vi "Bernards_2_2400.vi"() -> ()   [LabVIEW 2018]
uses:
  <vilib>/Utility/file.llb/Write Delimited Spreadsheet (string).vi
  <instrlib>/Keithley 24XX/Public/Data/Read (Single Point).vi
  <instrlib>/Keithley 24XX/Keithley 24XX.lvlib
  <vilib>/Analysis/NI_AALBase.lvlib
panel:
  in  "Auto (up)\nUser (down)":bool
  in  "User Selected":dbl[](array[numeric])=[-2e-08, -5e-08, -1e-07]
  in  "CC (on), CV (off)":bool
  out "Current (A) 2":dbl format="%.2e"
  out "error 8":string
  in  "Keithley 2401 (new)\nVISA resource #2 = 22":refnum<visa-resource-name>="GPIB0::22::INSTR"
  in  "Delay Gate (s) 2":dbl=60.0 format="%#.3g"
  in  "source/measure (V/I:0)":u16(ring)=1 items=["voltage/current", "current/voltage"]
  out "Setpoint Array":dbl[](array[numeric])=[-2e-08, -5e-08, -1e-07]
  in  "Measurement Speed (1 PLC)":dbl=1.0 format="%.2g"
  in  "Initial Gate Setting":dbl=1e-08 format="%#.3e"
  in  "Voltage Compliance Limit 2401 (V)":dbl=-0.95 format="%#.3f"
  in  "Current Compliance\nLimit 2401 (A)":dbl=0.10000000009313226
  in  "Delay Gate (s)":dbl=30.0 format="%#.3g"
  in  "Keithley 237 GPIB address":string="17"
  in  "Wait Time Btwn Keithley Readings (ms)":i32=30
  out "Time Btwn Iterations (ms)":i32
  out "Total Elapsed Time (ms)":i32
  out "# Avgs":i32
  out "Current (A)":dbl format="%.2e"
  in  "Total Measure Time (s)":dbl=210.0 format="%#.3g"
  in  "Drain Bias (V)":dbl=-0.6 format="%#.3g"
  in  "Current Compliance\nLimit (A)":dbl=0.5 format="%#.3e"
  in  "Keithley 2400 (old)\nVISA resource #1 = 24":refnum<visa-resource-name>="GPIB0::24::INSTR"
  in  "ApproximateTime Step (ms)":dbl=300.0 format="%#.3g"
  in  "Current Offset":dbl format="%^#_3e"
  out "I-t Measurement\nBy M. Ziffer 7/3/2014":cluster{dbl[], dbl[]}(graph)={[-2.0, -1.95, -1.9, -1.85, -1.8, -1.75, -1.7, -1.65, -1.6, -1.55, -1.5, -1.45, -1.4, -1.35, -1.2999999999999998, -1.25, -1.2, -1.15, -1.1, -1.0499999999999998, -1.0, -0.95, -0.8999999999999999, -0.8499999999999999, -0.7999999999999998, -0.75, -0.7, -0.6499999999999999, -0.5999999999999999, -0.5499999999999998, -0.5, -0.44999999999999996, -0.3999999999999999, -0.34999999999999987, -0.2999999999999998, -0.25, -0.19999999999999996, -0.1499999999999999, -0.09999999999999987, -0.04999999999999982, 0.0, 0.050000000000000266, 0.10000000000000009, 0.1499999999999999, 0.20000000000000018, 0.25, 0.30000000000000027, 0.3500000000000001, 0.40000000000000036, 0.4500000000000002, 0.5, 0.5500000000000003, 0.6000000000000001, 0.6500000000000004, 0.7000000000000002, 0.75, 0.8000000000000003, 0.8500000000000001, 0.9000000000000004, 0.9500000000000002, 1.0, 1.0500000000000003, 1.1, 1.1500000000000004, 1.2000000000000002, 1.25, 1.3000000000000003, 1.35, 1.4000000000000004, 1.4500000000000002, 1.5, 1.5500000000000003, 1.6, 1.6500000000000004, 1.7000000000000002, 1.75, 1.8000000000000003, 1.85, 1.9000000000000004, 1.9500000000000002, 2.0, 1.95, 1.9, 1.85, 1.8, 1.75, 1.7, 1.65, 1.6, 1.55, 1.5, 1.45, 1.4, 1.35, 1.2999999999999998, 1.25, 1.2, 1.15, 1.1, 1.0499999999999998, 1.0, 0.95, 0.8999999999999999, 0.8499999999999999, 0.7999999999999998, 0.75, 0.7, 0.6499999999999999, 0.5999999999999999, 0.5499999999999998, 0.5, 0.44999999999999996, 0.3999999999999999, 0.34999999999999987, 0.2999999999999998, 0.25, 0.19999999999999996, 0.1499999999999999, 0.09999999999999987, 0.04999999999999982, 0.0, -0.050000000000000266, -0.10000000000000009, -0.1499999999999999, -0.20000000000000018, -0.25, -0.30000000000000027, -0.3500000000000001, -0.40000000000000036, -0.4500000000000002, -0.5, -0.5500000000000003, -0.6000000000000001, -0.6500000000000004, -0.7000000000000002, -0.75, -0.8000000000000003, -0.8500000000000001, -0.9000000000000004, -0.9500000000000002, -1.0, -1.0500000000000003, -1.1, -1.1500000000000004, -1.2000000000000002, -1.25, -1.3000000000000003, -1.35, -1.4000000000000004, -1.4500000000000002, -1.5, -1.5500000000000003, -1.6, -1.6500000000000004, -1.7000000000000002, -1.75, -1.8000000000000003, -1.85, -1.9000000000000004, -1.9500000000000002, -2.0], [-0.9617289445307117, -0.9618513744908972, -0.9601574911889584, -0.9603488957746004, -0.9598860982876659, -0.9595594700613103, -0.9590290885663679, -0.9586886097902229, -0.9580144940757807, -0.9570474587019399, -0.9571418538143588, -0.9562287187728303, -0.9551771894828052, -0.9535572870291384, -0.9535421571112963, -0.9533114258642045, -0.9520938012261039, -0.9513117179729429, -0.9508812384355169, -0.9504840780921618, -0.9504173840793213, -0.9482281628421478, -0.9464640811713977, -0.9453356785488072, -0.9439408336230415, -0.9428695575652444, -0.9416178906119992, -0.9396031084275935, -0.9378375248899987, -0.9354517815949719, -0.9324159524550173, -0.928767917889437, -0.9245502864168607, -0.9203528467096396, -0.9146985405384399, -0.908595454304189, -0.9012966039381313, -0.8917361646028689, -0.8808115851751085, -0.8684870433493713, -0.853007079283089, -0.8360736418594031, -0.8154860511533626, -0.7920970894092216, -0.7641180332150388, -0.7294003786125389, -0.6854183749419586, -0.6263231964633708, -0.5399961516707377, -0.4044042921440459, -0.19129744134883978, 0.11936942255465804, 0.5420583260977958, 1.0996962734707192, 1.8318907919106253, 2.7834859177196174, 3.9948214605959804, 5.494887344369723, 7.293988211209965, 9.39251059714275, 11.765998658717283, 14.371720946722268, 17.153138293174568, 20.070768287470067, 23.082285540692517, 26.15604905590766, 29.26009131920428, 32.38734131897913, 35.54092126952808, 38.70923397757575, 41.89103456238207, 45.09512285116253, 48.318234786641504, 51.57411300669423, 54.84161623237131, 58.130390342544004, 61.4596508891188, 64.79419021952893, 68.17503711098149, 71.57587551887687, 75.0023346626475, 71.8977923333163, 68.72637799211101, 65.51757272894447, 62.2950059155054, 59.076872390492845, 55.84672949319313, 52.615591470047114, 49.383497814590335, 46.15858586388574, 42.93308596012382, 39.714879010509975, 36.494540522470736, 33.276879251143754, 30.087779593472593, 26.903443634933772, 23.758388169345494, 20.669969771208738, 17.671195580039395, 14.804861569698371, 12.12778391916459, 9.68736655227705, 7.528128139792144, 5.673530623057721, 4.128839936603901, 2.8787577310032053, 1.895544581260216, 1.1383875896205915, 0.5622048852612092, 0.12746496878202787, -0.18928305409978952, -0.4042961076690051, -0.5411369085387429, -0.6286316214282486, -0.6871327837574404, -0.7298882072135505, -0.7640718647157413, -0.7921132761963248, -0.8155779431543743, -0.8358809022810104, -0.8523300154596555, -0.8668520109778625, -0.8802307520791266, -0.8907705198464766, -0.8998007445608903, -0.9078572589377096, -0.9150023626386364, -0.9215738644543149, -0.925261336930741, -0.9288795566582202, -0.9332418679701618, -0.9352489739462505, -0.9376688708058178, -0.9394550911063516, -0.9405290371496502, -0.9430050037047499, -0.9440335043698243, -0.9453382929096107, -0.9473152502994113, -0.9474565926568992, -0.9494901203645137, -0.94896546821346, -0.9503187058651598, -0.9511280452203158, -0.9523093469306558, -0.9532668704811476, -0.9541692143312739, -0.9545545822386634, -0.955485183435348, -0.9561708134622656, -0.956805602515258, -0.9577699122788996, -0.9578049002139094, -0.9580356870856992, -0.958780001168953, -0.9592832934359943, -0.9588639388381576, -0.959203916992021, -0.9603773199952523, -0.9611007191920772, -0.9623172869609168]}
  in  "First bias settle (ms)":dbl=2000.0 format="%#.2f"
  out "Outputfile":path
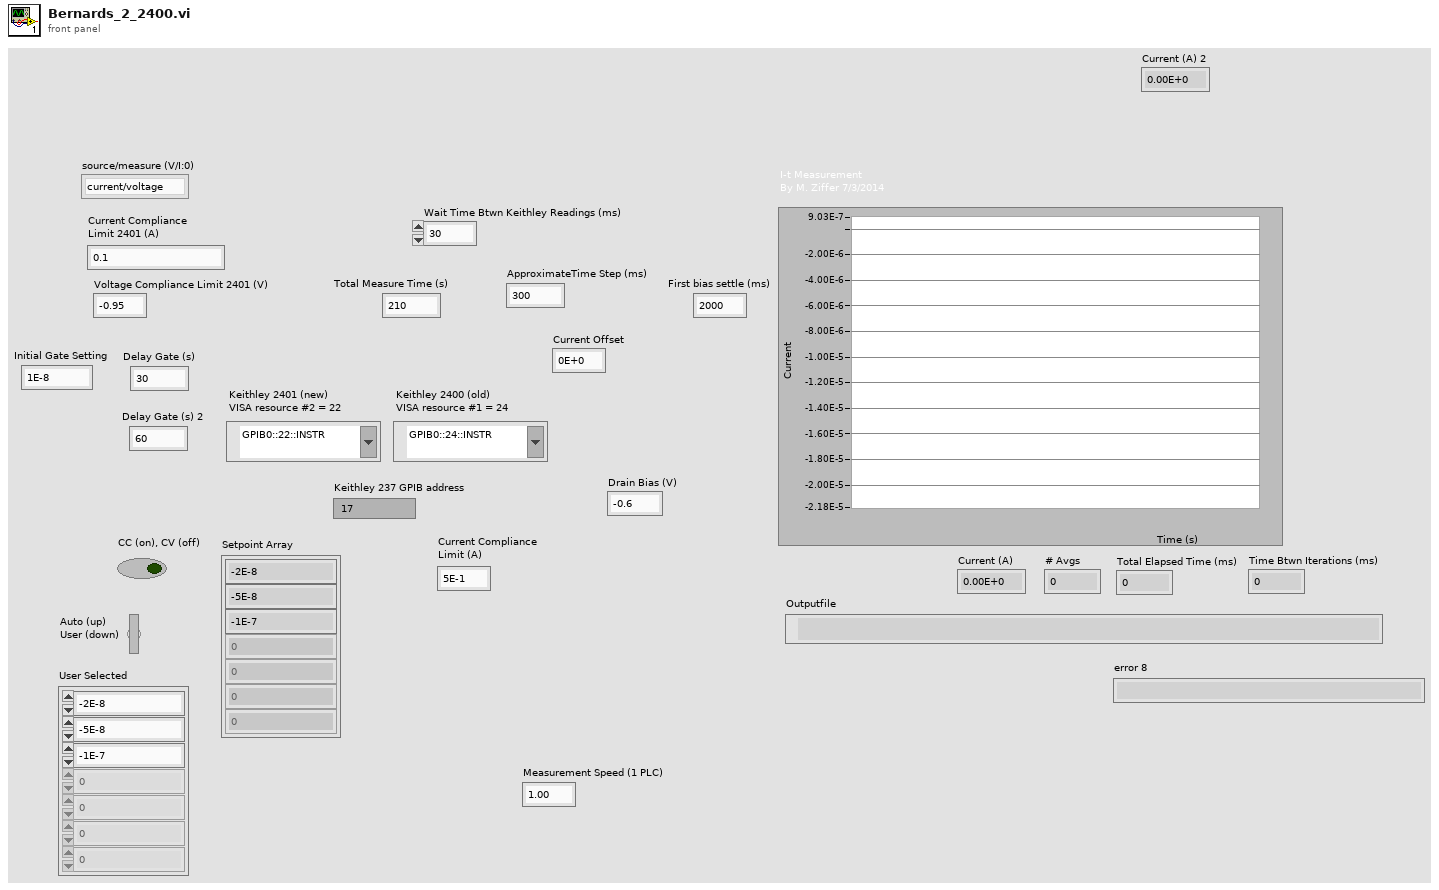
[diagram p1: front panel]
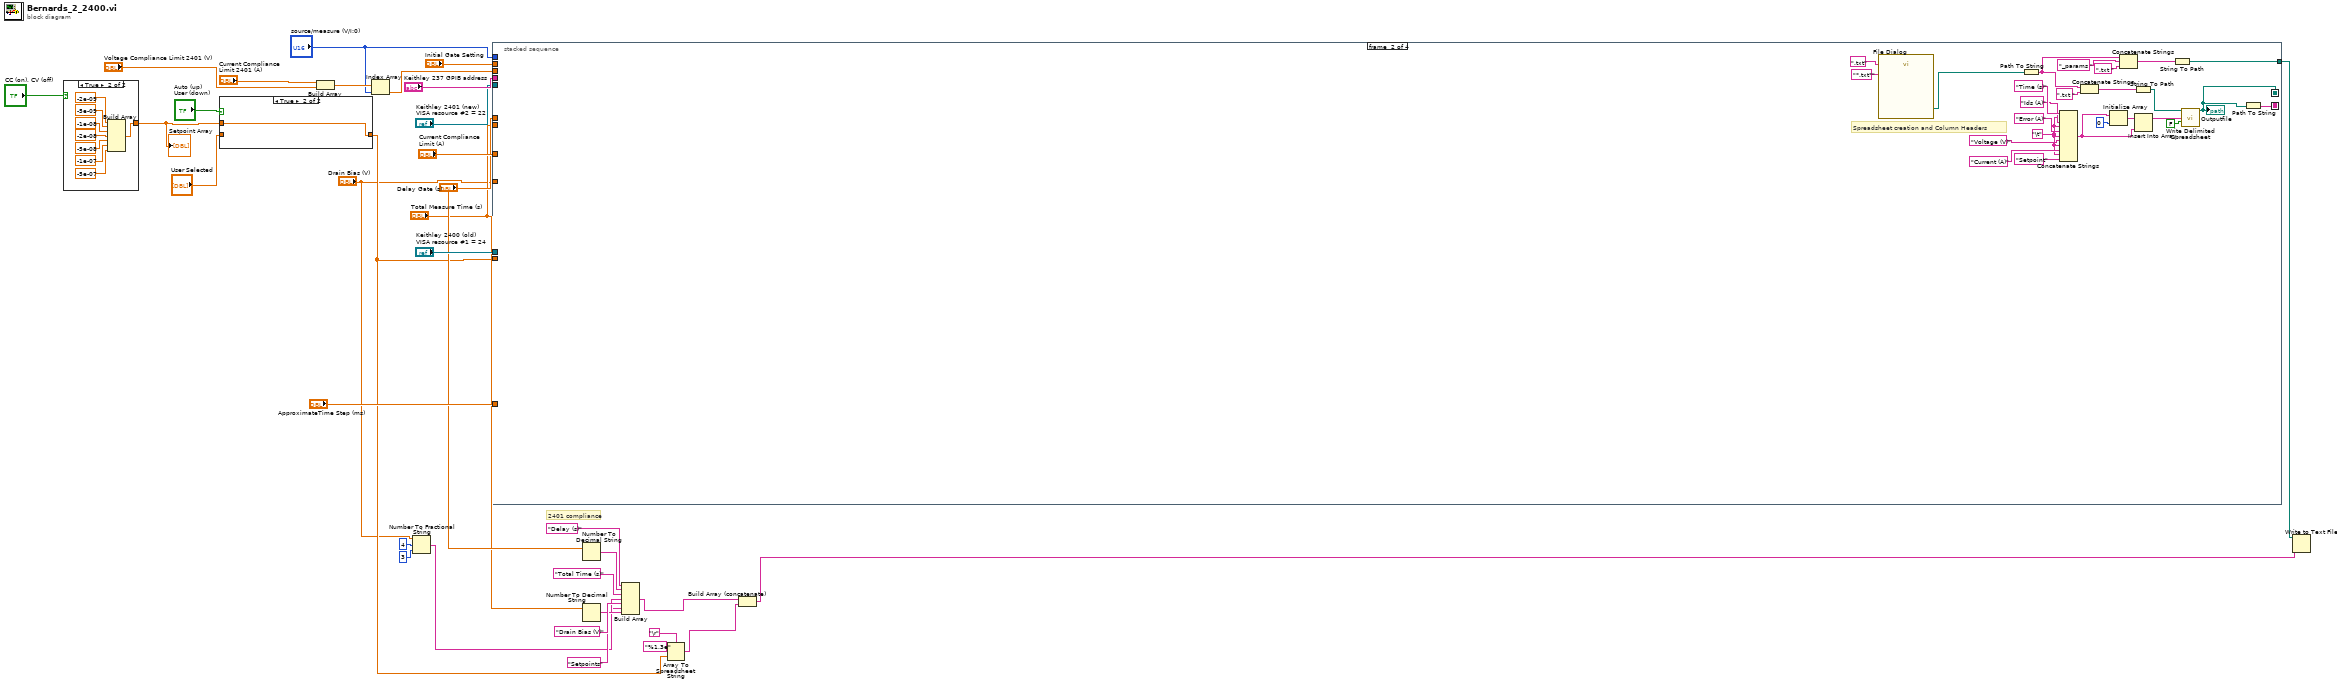
[diagram p0: block diagram]
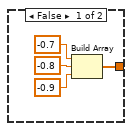
[diagram p3: hidden frame]
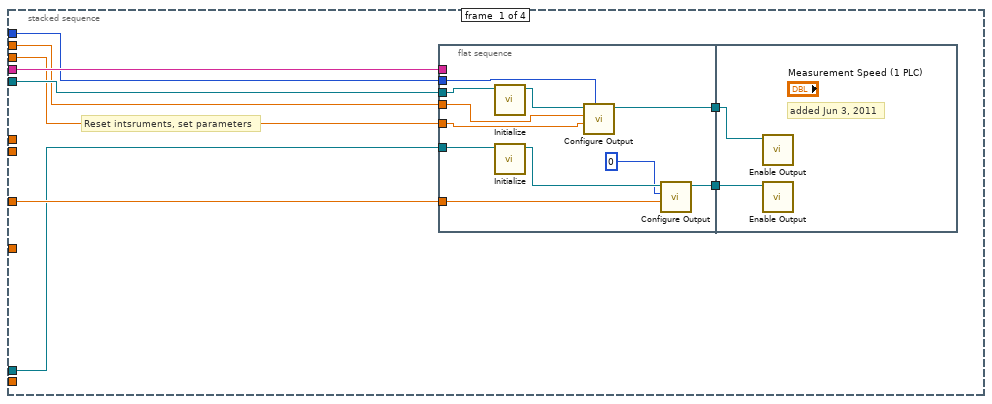
[diagram p4: hidden frame]
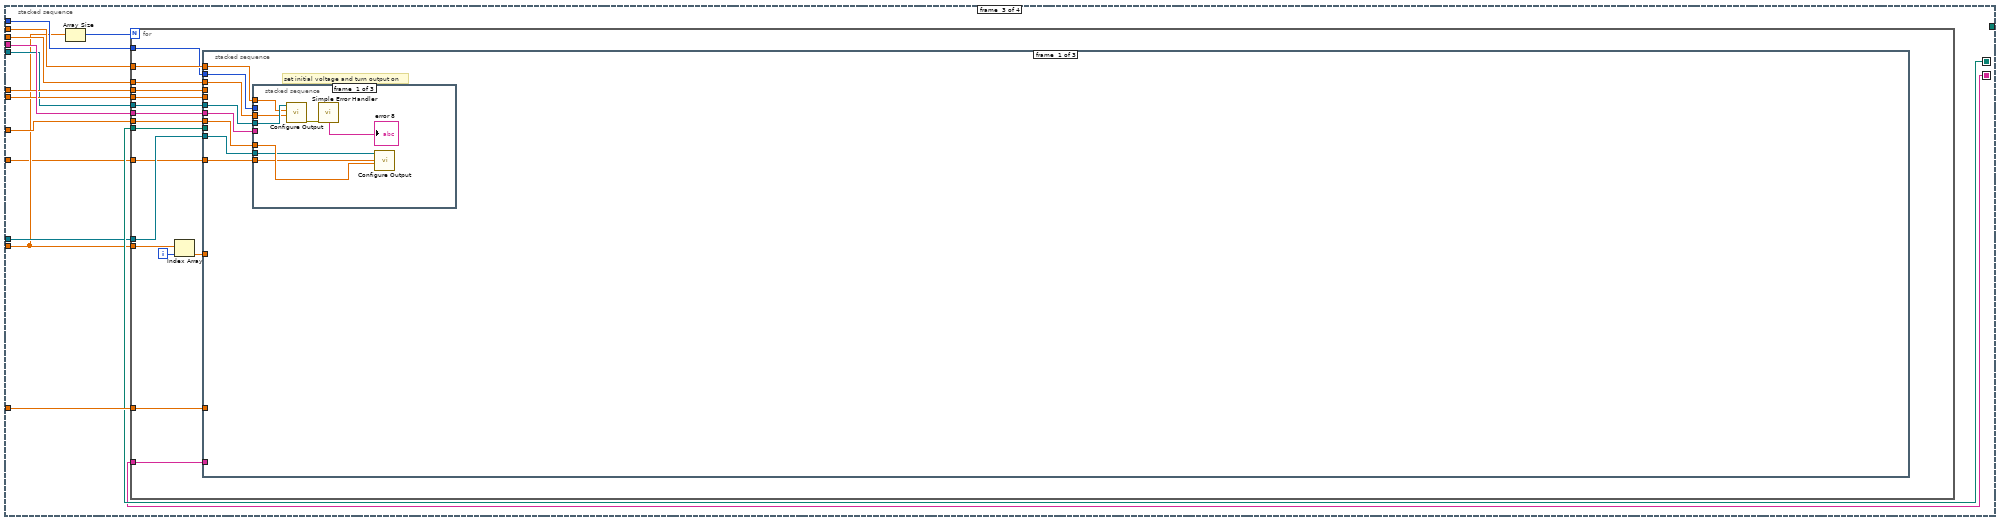
[diagram p5: hidden frame]
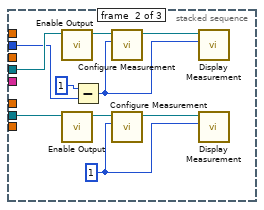
[diagram p6: hidden frame]
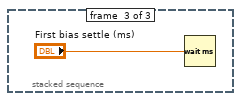
[diagram p7: hidden frame]
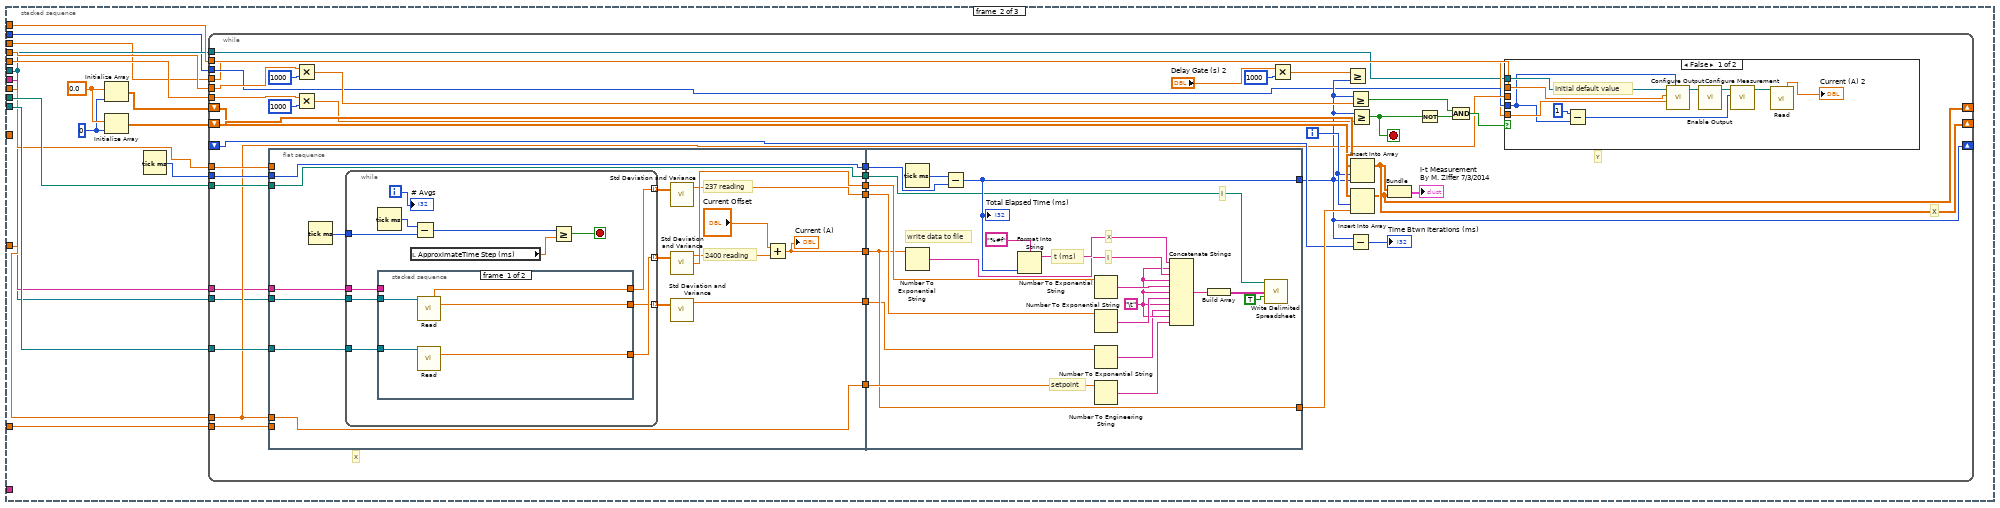
[diagram p8: hidden frame]
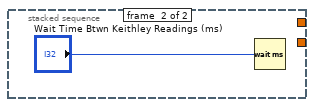
[diagram p9: hidden frame]
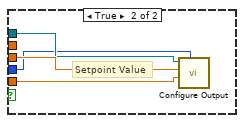
[diagram p10: hidden frame]
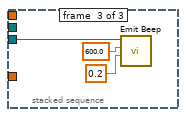
[diagram p11: hidden frame]
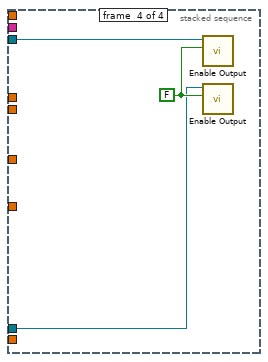
[diagram p12: hidden frame]
diagram:
  # "2401 compliance"
  n1 = case shown="True" "CC (on), CV (off)" {
    tunnel: [w38 w39] -> w17
    frame False {
      n2 = Build Array(-0.7, -0.8, -0.9) -> (w38:dbl[])
    }
    frame True {
      n3 = Build Array(-2e-09, -5e-09, -1e-08, -2e-08, -5e-08, -1e-07, -5e-07) -> (w39:dbl[])
    }
  }
  "Setpoint Array" <- w17
  n4 = case shown="True" "Auto (up)\nUser (down)" {
    tunnel: "User Selected" -> [w47 _]
    tunnel: w17 -> [_ w48]
    tunnel: [w47 w48] -> w16
    frame False {
    }
    frame True {
    }
  }
  n5 = Build Array("Current Compliance\nLimit 2401 (A)", "Voltage Compliance Limit 2401 (V)") -> (w24:dbl[])
  n6 = Index Array(array=w24, index="source/measure (V/I:0)") -> (element=w22:dbl)
  n7 = Number To Fractional String(number="Drain Bias (V)", width (-)=4, precision (6)=3) -> (F-format string=w3:string)  [unwired: 1 in]
  n8 = stacked-sequence {
    seq-local: [_ w76 _ _] -> [_ _ w109 _]
    seq-local: [_ w95 _ _] -> [_ _ w108 _]
    tunnel: "ApproximateTime Step (ms)" -> [_ _ w110 _]
    tunnel: "Keithley 2400 (old)\nVISA resource #1 = 24" -> [w56 _ w106 w284]
    tunnel: "Current Compliance\nLimit (A)" -> [w57 _ w107 _]
    tunnel: "Keithley 237 GPIB address" -> [w55 _ w104 _]
    tunnel: "Initial Gate Setting" -> [w51 _ w105 _]
    tunnel: "source/measure (V/I:0)" -> [w54 _ w99 _]
    tunnel: [_ w71 _ _] -> w30
    tunnel: "Delay Gate (s)" -> [_ _ w102 _]
    tunnel: "Total Measure Time (s)" -> [_ _ w101 _]
    tunnel: "Keithley 2401 (new)\nVISA resource #2 = 22" -> [w53 _ w100 w285]
    tunnel: w22 -> [w52 _ w98 _]
    tunnel: w16 -> [_ _ w97 _]
    tunnel: "Drain Bias (V)" -> [_ _ w96 _]
    frame #0 {
      # "Reset intsruments, set parameters"
      n9 = flat-sequence {
        tunnel: w56 -> [w67]
        tunnel: w57 -> [w63]
        tunnel: w55 -> [_]
        tunnel: w54 -> [w62]
        tunnel: w53 -> [w65]
        tunnel: w52 -> [w61]
        tunnel: w51 -> [w60]
        tunnel: [w68] -> w50
        tunnel: [w58] -> w49
        tunnel: w50 -> [w70]
        tunnel: w49 -> [w69]
        frame #0 {
          n10 = call <instrlib>:"Initialize.vi"("VISA resource name"=w65) -> ("VISA resource name out"=w64:refnum<visa-resource-name>)  [unwired: 9 in, 1 out]
          n11 = call <instrlib>:"Initialize.vi"("VISA resource name"=w67) -> ("VISA resource name out"=w66:refnum<visa-resource-name>)  [unwired: 9 in, 1 out]
          n12 = call <instrlib>:"Configure Output.vi"("Source Mode  (0: Voltage)"=w62, "Compliance  Level (0.1)"=w61, "Output Level (0)"=w60, "VISA resource name"=w64) -> ("VISA resource name out"=w58:refnum<visa-resource-name>)  [unwired: 2 in, 5 out]
          n13 = call <instrlib>:"Configure Output.vi"("Compliance  Level (0.1)"=w63, "Output Level (0)"=0, "VISA resource name"=w66) -> ("VISA resource name out"=w68:refnum<visa-resource-name>)  [unwired: 3 in, 5 out]
        }
        frame #1 {
          # "added Jun 3, 2011"
          n14 = call <instrlib>:"Enable Output.vi"("VISA resource name"=w69) -> ()  [unwired: 2 in, 9 out]
          n15 = call <instrlib>:"Enable Output.vi"("VISA resource name"=w70) -> ()  [unwired: 2 in, 9 out]
        }
      }
    }
    frame #1 {
      w78 = "\t"
      # "Spreadsheet creation and Column Headers"
      n16 = call "File Dialog"("default name"=".txt", "pattern (all files)"="*.txt*") -> ("selected path"=w82:path)  [unwired: 5 in, 8 out]
      n17 = Path To String(path=w82) -> (string=w73:string)
      n18 = Concatenate Strings("Time (s)", w78, "Ids (A)", w78, "Error (A)", w78, "Voltage (V)", w78, "Current (A)", w78, "Setpoint") -> (w93:string)
      n19 = Concatenate Strings(w73, ".txt " ("string")) -> (w81:string)
      n20 = Initialize Array(w93, 0 ("dimension size")) -> (w92:string[])
      n21 = Concatenate Strings(w73, "_params " ("string"), ".txt " ("string")) -> (w72:string)
      n22 = String To Path(string=w81) -> (path=w80:path)
      n23 = Insert Into Array(array=w92, new element=w93) -> (w85:string[])  [unwired: 1 in]
      n24 = String To Path(string=w72) -> (path=w71:path)
      n25 = call-poly <vilib>:"Write Delimited Spreadsheet.vi"("file path (dialog if empty)"=w80, "1D data"=w85, "append to file? (new file:F)"=FALSE) -> ("new file path (Not A Path if cancelled)"=w76:path)  [unwired: 11 in, 1 out]
      "Outputfile" <- w76
      n26 = Path To String(path=w76) -> (string=w95:string)
    }
    frame #2 {
      n27 = Array Size(array=w97) -> (size(s)=w103:i32)
      n28 = for {
        N: w103 -> [_]
        tunnel: w110 -> [w126]
        tunnel: w109 -> [w125]
        tunnel: w108 -> [w124]
        tunnel: w107 -> [w123]
        tunnel: w106 -> [w122]
        tunnel: w105 -> [w121]
        tunnel: w104 -> [w115]
        tunnel: w97 -> [w120]
        tunnel: w102 -> [w117]
        tunnel: w101 -> [w116]
        tunnel: w100 -> [w114]
        tunnel: w99 -> [w113]
        tunnel: w98 -> [w112]
        tunnel: w96 -> [w111]
        i -> [w118]
        n29 = Index Array(array=w120, index=w118) -> (element=w119:dbl)
        n30 = stacked-sequence {
          tunnel: w126 -> [_ w163 _]
          tunnel: w125 -> [_ w170 _]
          tunnel: w124 -> [_ _ _]
          tunnel: w123 -> [w134 w164 _]
          tunnel: w122 -> [w133 w165 w283]
          tunnel: w121 -> [w130 w161 _]
          tunnel: w115 -> [w132 w157 _]
          tunnel: w119 -> [_ w160 _]
          tunnel: w117 -> [_ w159 _]
          tunnel: w116 -> [_ w158 _]
          tunnel: w114 -> [w131 w156 _]
          tunnel: w113 -> [w129 w155 _]
          tunnel: w112 -> [w128 w154 _]
          tunnel: w111 -> [w127 _ _]
          frame #0 {
            # "set initial voltage and turn output on"
            n31 = stacked-sequence {
              tunnel: w133 -> [w141 w152 _]
              tunnel: w134 -> [w142 _ _]
              tunnel: w132 -> [_ _ _]
              tunnel: w131 -> [w140 w151 _]
              tunnel: w130 -> [w139 _ _]
              tunnel: w129 -> [_ w147 _]
              tunnel: w128 -> [w138 _ _]
              tunnel: w127 -> [w135 _ _]
              frame #0 {
                n32 = call <instrlib>:"Configure Output.vi"("Compliance  Level (0.1)"=w138, "Output Level (0)"=w139, "VISA resource name"=w140) -> ("error out"=w137:errorcluster)  [unwired: 3 in, 5 out]
                n33 = call <vilib>:"Simple Error Handler.vi"("error in (no error)"=w137) -> ("message"=→"error 8":string)  [unwired: 1 in, 7 out]
                n34 = call <instrlib>:"Configure Output.vi"("Compliance  Level (0.1)"=w142, "Output Level (0)"=w135, "VISA resource name"=w141) -> ()  [unwired: 3 in, 6 out]
              }
              frame #1 {
                w143 = 1
                n35 = call <instrlib>:"Enable Output.vi"("VISA resource name"=w151) -> ("VISA resource name out"=w150:refnum<visa-resource-name>)  [unwired: 2 in, 8 out]
                n36 = call <instrlib>:"Enable Output.vi"("VISA resource name"=w152) -> ("VISA resource name out"=w149:refnum<visa-resource-name>)  [unwired: 2 in, 8 out]
                n37 = Subtract(x=1, y=w147) -> (x-y=w144:i32)
                n38 = call <instrlib>:"Configure Measurement.vi"("Function (0: Volts)"=w144, "VISA resource name"=w150) -> ("VISA resource name out"=w145:refnum<visa-resource-name>)  [unwired: 8 in, 1 out]
                n39 = call <instrlib>:"Configure Measurement.vi"("Function (0: Volts)"=w143, "VISA resource name"=w149) -> ("VISA resource name out"=w146:refnum<visa-resource-name>)  [unwired: 8 in, 1 out]
                n40 = call <instrlib>:"Display Measurement.vi"("Displayed Measurement (0: Voltage)"=w144, "VISA resource name"=w145) -> ()  [unwired: 8 in, 2 out]
                n41 = call <instrlib>:"Display Measurement.vi"("Displayed Measurement (0: Voltage)"=w143, "VISA resource name"=w146) -> ()  [unwired: 8 in, 2 out]
              }
              frame #2 {
                n42 = Wait (ms)(milliseconds to wait="First bias settle (ms)") -> ()  [unwired: 1 out]
              }
            }
          }
          frame #1 {
            w166 = 0
            w167 = 0.0
            n43 = Initialize Array(w167, w166) -> (w168:dbl[])
            n44 = Initialize Array(w167, w166) -> (w169:dbl[])
            n45 = Tick Count (ms)() -> (millisecond timer value=w162:u32)
            n46 = while {
              shift-left: w168 -> [w209]
              shift-right: [w204] -> _
              shift-left: w169 -> [w210]
              shift-right: [w206] -> _
              tunnel: w170 -> [w211]
              tunnel: w165 -> [w208]
              tunnel: w164 -> [w207]
              tunnel: w163 -> [w202]
              tunnel: w162 -> [w197]
              shift-right: [w179] -> _
              shift-left: _ -> [w201]
              tunnel: w157 -> [w188]
              tunnel: w161 -> [w194]
              tunnel: w160 -> [w189]
              tunnel: w159 -> [w176]
              tunnel: w158 -> [w175]
              tunnel: w156 -> [w174]
              tunnel: w156 -> [w171]
              tunnel: w155 -> [w173]
              tunnel: w154 -> [w172]
              i -> [w203]
              stop <- w193 stop-if-true
              # "X"
              # "X"
              # "Y"
              n47 = flat-sequence {
                tunnel: w211 -> [w222]
                tunnel: [w222] -> w187
                tunnel: w208 -> [w216]
                tunnel: w207 -> [_]
                tunnel: w202 -> [_]
                tunnel: w197 -> [w221]
                tunnel: [w221] -> w186
                tunnel: w189 -> [w220]
                tunnel: [w220] -> w185
                tunnel: w188 -> [w223]
                tunnel: [w228] -> w184
                tunnel: [w224] -> w183
                tunnel: [w219] -> w182
                tunnel: [w218] -> w177
                tunnel: w174 -> [w217]
                tunnel: [w252] -> w205
                tunnel: w187 -> [w247]
                tunnel: w186 -> [w259]
                tunnel: [w258] -> w179
                tunnel: w185 -> [w255]
                tunnel: w184 -> [w261]
                tunnel: w183 -> [w252]
                tunnel: w182 -> [w254]
                tunnel: w177 -> [w248]
                frame #0 {
                  # "2400 reading"
                  # "237 reading"
                  n48 = Tick Count (ms)() -> (millisecond timer value=w225:u32)
                  n49 = while {
                    tunnel: w225 -> [w239]
                    tunnel: w223 -> [w234]
                    tunnel: w217 -> [w233]
                    tunnel: w216 -> [w232]
                    tunnel: [w231] -> w215 mode=indexing
                    tunnel: [w230] -> w214 mode=indexing
                    tunnel: [w229] -> w213 mode=indexing
                    i -> [w240]
                    stop <- w237 stop-if-true
                    n50 = Tick Count (ms)() -> (millisecond timer value=w236:u32)
                    n51 = stacked-sequence {
                      tunnel: w234 -> [_ _]
                      tunnel: w233 -> [w244 _]
                      tunnel: w232 -> [w245 _]
                      tunnel: [w243 _] -> w231
                      tunnel: [w242 _] -> w230
                      tunnel: [w241 _] -> w229
                      frame #0 {
                        n52 = call-poly <instrlib>:"Read.vi"("VISA resource name"=w244) -> ("Voltage"=w242:sgl, "Current"=w241:sgl)  [unwired: 8 in, 5 out]
                        n53 = call-poly <instrlib>:"Read.vi"("VISA resource name"=w245) -> ("Current"=w243:sgl)  [unwired: 8 in, 6 out]
                      }
                      frame #1 {
                        n54 = Wait (ms)(milliseconds to wait="Wait Time Btwn Keithley Readings (ms)") -> ()  [unwired: 1 out]
                      }
                    }
                    n55 = local read "ApproximateTime Step (ms)"() -> (w235:dbl)
                    n56 = Subtract(x=w236, y=w239) -> (x-y=w238:u32)
                    n57 = Greater Or Equal?(x=w238, y=w235) -> (x >= y?=w237:bool)
                    "# Avgs" <- w240
                  }
                  n58 = call <vilib>:"Std Deviation and Variance.vi"("X"=w214) -> ("mean"=w219:dbl)  [unwired: 1 in, 2 out]
                  n59 = call <vilib>:"Std Deviation and Variance.vi"("X"=w215) -> ("mean"=w227:dbl, "standard deviation"=w228:dbl)  [unwired: 1 in, 1 out]
                  n60 = call <vilib>:"Std Deviation and Variance.vi"("X"=w213) -> ("mean"=w218:dbl)  [unwired: 1 in, 2 out]
                  n61 = Add(x="Current Offset", y=w227) -> (x+y=w224:dbl)
                  "Current (A)" <- w224
                }
                frame #1 {
                  w250 = "\t"
                  # "setpoint"
                  # "I"
                  # "I"
                  # "t (ms)"
                  # "write data to file"
                  # "X"
                  n62 = Tick Count (ms)() -> (millisecond timer value=w260:u32)
                  n63 = Number To Exponential String(number=w252) -> (E-format string=w264:string)  [unwired: 3 out]
                  n64 = Subtract(x=w260, y=w259) -> (x-y=w258:u32)
                  "Total Elapsed Time (ms)" <- w258
                  n65 = Format Into String(format string="%#f", w258) -> (resulting string=w265:string)  [unwired: 2 in, 1 out]
                  n66 = Number To Exponential String(number=w261) -> (E-format string=w262:string)  [unwired: 3 out]
                  n67 = Number To Exponential String(number=w254) -> (E-format string=w253:string)  [unwired: 3 out]
                  n68 = Number To Exponential String(number=w248) -> (E-format string=w249:string)  [unwired: 3 out]
                  n69 = Number To Engineering String(4:w255) -> (0:w251:string)  [unwired: 3 in]
                  n70 = Concatenate Strings(w265, w250, w264, w250, w262, w250, w253, w250, w249, w250, w251) -> (w263:string)
                  n71 = Build Array(w263) -> (w257:string[])
                  n72 = call-poly <vilib>:"Write Delimited Spreadsheet.vi"("file path (dialog if empty)"=w247, "1D data"=w257, "append to file? (new file:F)"=TRUE) -> ()  [unwired: 11 in, 2 out]
                }
              }
              n73 = Multiply(x=w176, y=1000) -> (x*y=w196:dbl)
              n74 = Multiply(x=w175, y=1000) -> (x*y=w198:dbl)
              n75 = Multiply(x="Delay Gate (s) 2", y=1000) -> (x*y=w178:dbl)
              n76 = Greater Or Equal?(x=w178, y=w179) -> ()  [unwired: 1 out]
              n77 = Greater Or Equal?(x=w179, y=w196) -> (x >= y?=w191:bool)
              n78 = Subtract(x=w179, y=w201) -> (x-y=→"Time Btwn Iterations (ms)":u32)
              n79 = Greater Or Equal?(x=w179, y=w198) -> (x >= y?=w193:bool)
              n80 = Insert Into Array(array=w210, index=w203, new element=w179) -> (w206:dbl[])
              n81 = Insert Into Array(array=w209, index=w203, new element=w205) -> (w204:dbl[])
              n82 = Bundle(w206, w204) -> (→"I-t Measurement\nBy M. Ziffer 7/3/2014":cluster{dbl[], dbl[]})  [unwired: 1 out]
              n83 = Not(x=w193) -> (.not. x?=w192:bool)
              n84 = And(x=w191, y=w192) -> (x .and. y?=w190:bool)
              n85 = case shown="False" w190 {
                tunnel: w194 -> [w276 _]
                tunnel: w189 -> [_ w280]
                tunnel: w171 -> [w275 w279]
                tunnel: w173 -> [w268 w278]
                tunnel: w172 -> [w274 w277]
                frame False {
                  # "Initial default value"
                  n86 = Subtract(x=1, y=w268) -> (x-y=w267:i32)
                  n87 = call <instrlib>:"Configure Output.vi"("Source Mode  (0: Voltage)"=w268, "Compliance  Level (0.1)"=w274, "Output Level (0)"=w276, "VISA resource name"=w275) -> ("VISA resource name out"=w271:refnum<visa-resource-name>)  [unwired: 2 in, 5 out]
                  n88 = call <instrlib>:"Enable Output.vi"("VISA resource name"=w271) -> ("VISA resource name out"=w270:refnum<visa-resource-name>)  [unwired: 9 in, 1 out]
                  n89 = call <instrlib>:"Configure Measurement.vi"("Function (0: Volts)"=w267, "VISA resource name"=w270) -> ("VISA resource name out"=w269:refnum<visa-resource-name>)  [unwired: 8 in, 1 out]
                  n90 = call-poly <instrlib>:"Read.vi"("VISA resource name"=w269) -> ("Voltage"=→"Current (A) 2":sgl)  [unwired: 8 in, 6 out]
                }
                frame True {
                  # "Setpoint Value"
                  n91 = call <instrlib>:"Configure Output.vi"("Source Mode  (0: Voltage)"=w278, "Compliance  Level (0.1)"=w277, "Output Level (0)"=w280, "VISA resource name"=w279) -> ()  [unwired: 2 in, 6 out]
                }
              }
            }
          }
          frame #2 {
            n92 = call <instrlib>:"Emit Beep.vi"("Beep Duration (.25 s)"=0.2, "Beep Frequency (300)"=600.0, "VISA resource name"=w283) -> ()  [unwired: 7 in, 2 out]
          }
        }
      }
    }
    frame #3 {
      w286 = FALSE
      n93 = call <instrlib>:"Enable Output.vi"("Enable Output (T: Enable)"=w286, "VISA resource name"=w285) -> ()  [unwired: 8 in, 2 out]
      n94 = call <instrlib>:"Enable Output.vi"("Enable Output (T: Enable)"=w286, "VISA resource name"=w284) -> ()  [unwired: 8 in, 2 out]
    }
  }
  n95 = Number To Decimal String(number="Delay Gate (s)") -> (decimal integer string=w10:string)  [unwired: 1 in]
  n96 = Number To Decimal String(number="Total Measure Time (s)") -> (decimal integer string=w9:string)  [unwired: 1 in]
  n97 = Build Array("Delay (s)", w10, "Total Time (s)", w9, "Drain Bias (V)", w3, "Setpoints") -> (w7:string[])
  n98 = Array To Spreadsheet String(delimiter (Tab)="\r", array=w16, 3:"%1.3e") -> (spreadsheet string=w6:string)
  n99 = Build Array (concatenate)(w7, w6) -> (w5:string[])
  n100 = Write to Text File(file (use dialog)=w30, text=w5) -> ()  [unwired: 2 in, 3 out]
